vi "SWITCH Clear Data Buffer.vi"(8 "error in (no error)":errorcluster, 10 "Message Data":variant, 11 "Data Cluster in":T1={"Tango HW"={"VISA resource"="101:110", "Baud Rate (115200)"=0, "lAnInterfaceType"=0, "bAShowProt"=0}, "Writer Queue"=refnum, "Status"=FALSE, "Abs Position"=[], "Axis Velocity"={"dX"=0.0, "dY"=0.0, "dZ"=0.0, "dA"=0.0}, "acceleration "=0.0, "Z direction"=enum."Up", "Position Mode"="", "plLSID"=0}) -> (0 "error out":errorcluster, 3 "Data Cluster out":T1={"Tango HW"={"VISA resource"="101:110", "Baud Rate (115200)"=0, "lAnInterfaceType"=0, "bAShowProt"=0}, "Writer Queue"=refnum, "Status"=FALSE, "Abs Position"=[], "Axis Velocity"={"dX"=0.0, "dY"=0.0, "dZ"=0.0, "dA"=0.0}, "acceleration "=0.0, "Z direction"=enum."Up", "Position Mode"="", "plLSID"=0})   [LabVIEW 2020, in "MOTOR.lvlib"]
uses:
  MOTOR.lvlib
  support/Message Queue/Message Cluster.ctl
  support/Message Queue/Message Queue.lvlib
  support/HW Message Cluster.ctl
  PS Hardware Configuration.ctl
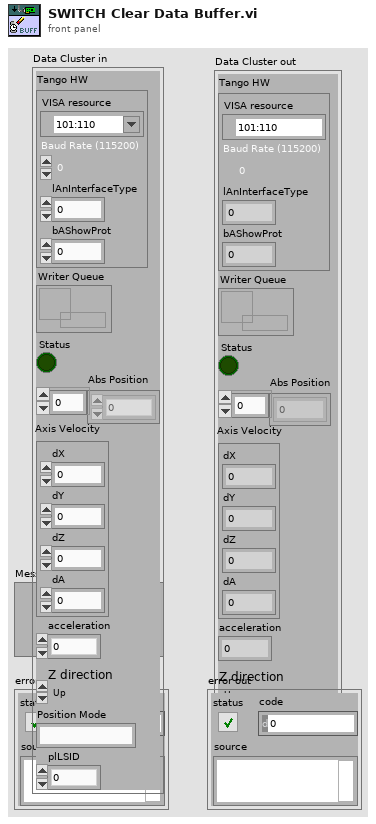
[diagram p1: front panel]
types:
  T1 = typedef "MOTOR.lvlib/PS Hardware Configuration.ctl" = cluster{"Tango HW":cluster{"VISA resource":refnum<visa-resource-name>, "Baud Rate (115200)":i32, "lAnInterfaceType":i32, "bAShowProt":i32}, "Writer Queue":refnum<queue>, "Status":bool, "Abs Position":i32[], "Axis Velocity":cluster{"dX":dbl, "dY":dbl, "dZ":dbl, "dA":dbl}, "acceleration ":dbl, "Z direction":enum16{"Up", "Down"}, "Position Mode":string, "plLSID":i32}
  T2 = typedef "Message Queue.lvlib/HW Message Cluster.ctl" = cluster{"Writer Queue":refnum<queue>, "Writer Data":T3}
  T3 = typedef "Message Queue.lvlib/Message Cluster.ctl" = cluster{"Message":string, "Message Data":variant}
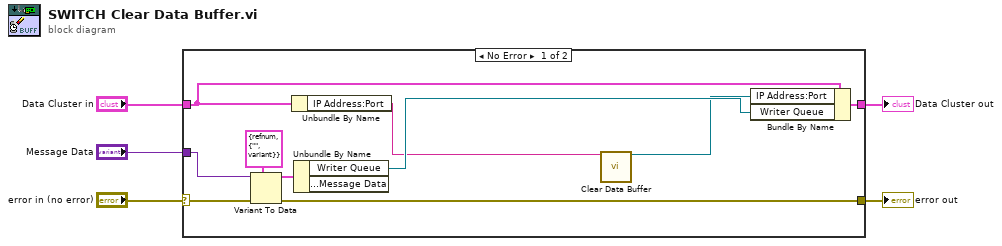
[diagram p0: block diagram]
diagram:
  n1 = case shown="No Error" "error in (no error)" {
    selector: "error in (no error)" -> [w12 w16]
    tunnel: "Message Data" -> [w10 _]
    tunnel: [w15 w17] -> w4
    tunnel: "Data Cluster in" -> [w14 w17]
    tunnel: [w11 w16] -> w2
    frame No Error {
      n2 = Variant To Data(error in=w12, type=T2 {"Writer Queue"=refnum, "Writer Data"={"Message"="", "Message Data"=variant}}, Variant=w10) -> (data=w13:T2, error out=w11:errorcluster)
      n3 = Unbundle By Name(w14) -> ("IP Address:Port"=w7:string)
      n4 = Unbundle By Name(w13) -> ("Writer Queue"=w9:refnum<queue>)  [unwired: 1 out]
      n5 = call <instrlib>:"Clear Data Buffer.vi"("VISA resource name"=w7) -> ("VISA resource name out"=w6:refnum<visa-resource-name>)  [unwired: 13 in, 1 out]
      n6 = Bundle By Name(cluster=w14, "IP Address:Port"=w6, "Writer Queue"=w9) -> (w15:T1)
    }
    frame Error {
    }
  }
  "Data Cluster out" <- w4
  "error out" <- w2
